vi "NewGPS.vi"(10 "Input lat, long, dev":dbl[](array[numeric]), 11 "GPS Com Port":refnum<visa-resource-name>="ASRL14::INSTR") -> (3 "Output lat, long, dev":dbl[](array[numeric]))   [LabVIEW 2014]
panel:
  # "Inputs:"
  # "Outputs:"
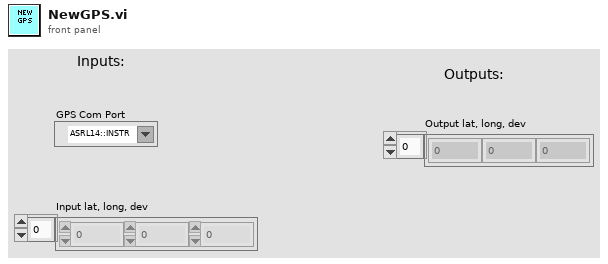
[diagram p1: front panel]
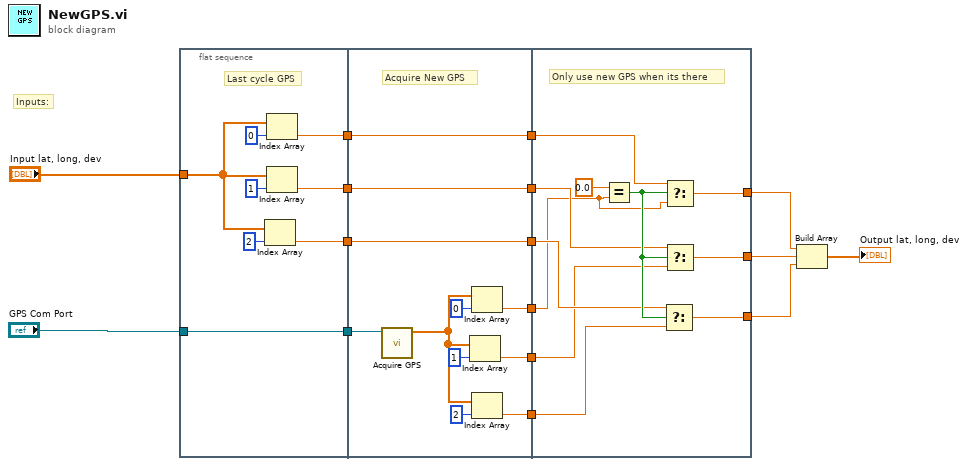
[diagram p0: block diagram]
diagram:
  # "Inputs:"
  n1 = flat-sequence {
    tunnel: "GPS Com Port" -> [w24]
    tunnel: [w24] -> w15
    tunnel: "Input lat, long, dev" -> [w23]
    tunnel: [w19] -> w10
    tunnel: [w18] -> w8
    tunnel: [w17] -> w6
    tunnel: w15 -> [w35]
    tunnel: [w33] -> w13
    tunnel: [w32] -> w12
    tunnel: [w31] -> w11
    tunnel: w10 -> [w30]
    tunnel: [w30] -> w9
    tunnel: w8 -> [w29]
    tunnel: [w29] -> w7
    tunnel: w6 -> [w28]
    tunnel: [w28] -> w5
    tunnel: w13 -> [w41]
    tunnel: w12 -> [w40]
    tunnel: w11 -> [w39]
    tunnel: w9 -> [w44]
    tunnel: w7 -> [w43]
    tunnel: w5 -> [w42]
    tunnel: [w38] -> w4
    tunnel: [w37] -> w3
    tunnel: [w36] -> w2
    frame #0 {
      # "Last cycle GPS"
      n2 = Index Array(array=w23, index=2) -> (element=w17:dbl)
      n3 = Index Array(array=w23, index=0) -> (element=w19:dbl)
      n4 = Index Array(array=w23, index=1) -> (element=w18:dbl)
    }
    frame #1 {
      # "Acquire New GPS"
      n5 = call "Acquire GPS.vi"("GPS COM Port"=w35) -> ("Lat, long, dev output"=w34:dbl[])  [unwired: 10 in]
      n6 = Index Array(array=w34, index=1) -> (element=w32:dbl)
      n7 = Index Array(array=w34, index=0) -> (element=w33:dbl)
      n8 = Index Array(array=w34, index=2) -> (element=w31:dbl)
    }
    frame #2 {
      # "Only use new GPS when its there"
      n9 = Equal?(x=0.0, y=w41) -> (x = y?=w46:bool)
      n10 = Select(t=w42, s=w46, f=w39) -> (s? t:f=w36:dbl)
      n11 = Select(t=w44, s=w46, f=w41) -> (s? t:f=w38:dbl)
      n12 = Select(t=w43, s=w46, f=w40) -> (s? t:f=w37:dbl)
    }
  }
  n13 = Build Array(w4, w3, w2) -> (→"Output lat, long, dev":dbl[])
